vi "GetAll.vi"() -> (2 "Added":refnum<user-event>, 3 "Modules":T1[](array[typedef]))   [LabVIEW 2024, in "FGVWithEventTrace.lvclass"]
uses:
  FGVWithEventTrace.lvclass
  DebugTraceHandle/StartArgs.ctl
  Command.ctl
  DebugTraceHandle/DebugTraceHandle.lvclass
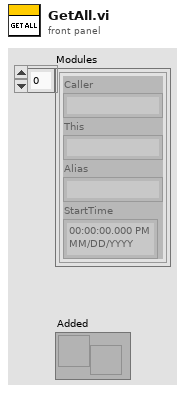
[diagram p1: front panel]
types:
  T1 = typedef "DebugTraceHandle.lvclass/StartArgs.ctl" = cluster{"Caller":string, "This":string, "Alias":string, "StartTime":timestamp}
  T2 = typedef "FGVWithEventTrace.lvclass/Command.ctl" = enum16{"Add", "Get", "Remove", "Clear"}
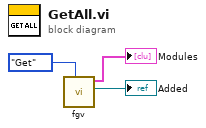
[diagram p0: block diagram]
diagram:
  n1 = call "fgv.vi"("Command"=Command."Get") -> ("Added"=→"Added":refnum<user-event>, "Modules"=→"Modules":T1[])  [unwired: 9 in]
